vi "Memory.Pointer.Allocate Filled Byte Array.vi"(8 "error in (no error)":errorcluster, 11 "pointer in":refnum<class "Memory.Pointer.lvclass">) -> (0 "error out":errorcluster, 2 "filled byte array":u8[](array[numeric]) format="%02x", 3 "pointer out":refnum<class "Memory.Pointer.lvclass">)   [LabVIEW 2016, in "Memory.lvlib" / "Memory.Pointer.lvclass"]
uses:
  Memory.Pointer.lvclass
  Memory.Pointer.lvclass/Memory.Pointer.ctl
  Memory.Pointer.Read.Safe.1D.U8.vi
  Memory.Pointer.Get Size.vi
  Memory.Pointer.Read.Unsafe.1D.U8.vi
  Memory.Pointer.Parameter Check.Null Pointer.vi
  Memory.Pointer.Parameter Check.Subset.Power of 2.vi
  Memory.Pointer.Get Address.vi
  Memory.Pointer.Errors.vi
  Memory.Pointer.Errors.Null Pointer.vi
  Memory.Pointer.Errors.Out of Bounds.vi
  VIs/Memory.Count to Size.Power of 2.vi
  Memory.Pointer.Errors.Create Error.vi
  Submodules/SEH/Source/VIs/Static Error Handling.Source Buffer.Write.String.vi
  Memory.Pointer.Errors.Write Pointer Size.vi
  Submodules/SEH/Source/VIs/Static Error Handling.Source Buffer.Write.Numeric.Scalar.Base10.vi
  Submodules/SEH/Source/VIs/Static Error Handling.Source Buffer.Write.Numeric.Scalar.Base10 (U64).vi
  Submodules/SEH/Source/VIs/Static Error Handling.Error Cluster Constant.vi
  Submodules/SEH/Source/VIs/Static Error Handling.Error Cluster Constant (256B).vi
  Submodules/SEH/Source/VIs/Static Error Handling.Parameters.Status.Set.vi
  Submodules/SEH/Source/VIs/Static Error Handling.Parameters.Code.Set.vi
  Submodules/SEH/Source/VIs/Static Error Handling.Parameters.VI Source.Set.vi
  Constants/Memory.Constants.vi
  Constants/Memory.Constants.Library Name.vi
  Memory.Pointer.Errors.Get Info.vi
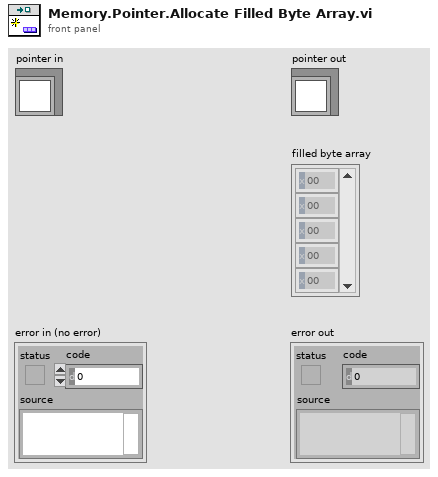
[diagram p1: front panel]
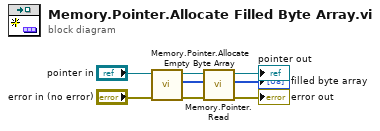
[diagram p0: block diagram]
diagram:
  n1 = call "Memory.Pointer.Allocate Empty Byte Array.vi"("error in (no error)"="error in (no error)", "pointer in"="pointer in") -> ("error out"=w2:errorcluster, "empty byte array"=w4:u8[], "pointer out"=w6:refnum<class "Memory.Pointer.lvclass">)  [unwired: 7 in]
  n2 = call-poly "Memory.Pointer.Read.vi"("error in (no error)"=w2, "buffer in"=w4, "pointer in"=w6) -> ("error out"=→"error out":errorcluster, "buffer out"=→"filled byte array":u8[], "pointer out"=→"pointer out":refnum<class "Memory.Pointer.lvclass">)  [unwired: 5 in, 1 out]
